vi "CICLO4.vi"() -> ()   [LabVIEW 2013]
panel:
  out "SUMA150":dbl
  out "Contador":dbl
  out "Velocidad Promedio":dbl
  out "Velocidad":dbl(knob) scale=0.0..220.0
  # "GENERAR 10 PRUEBA DE VELOCIDAD\nLUEGO SUMAR LAS VELOCIDADES \nMAYORES A 150 Y OBTENER SU PROMEDIO"
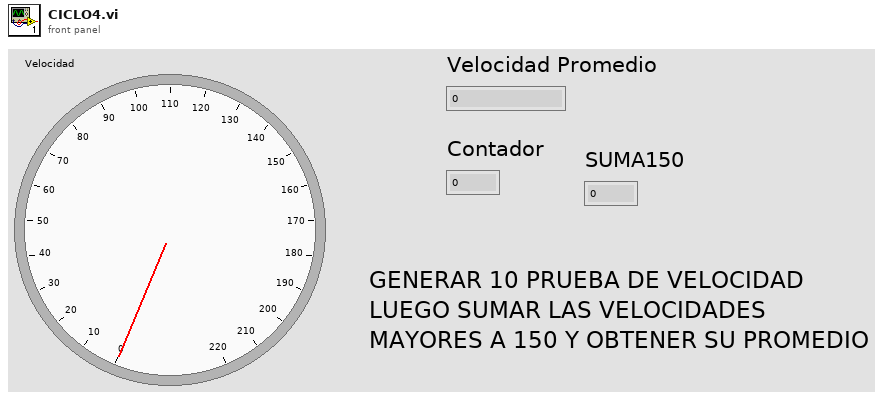
[diagram p1: front panel]
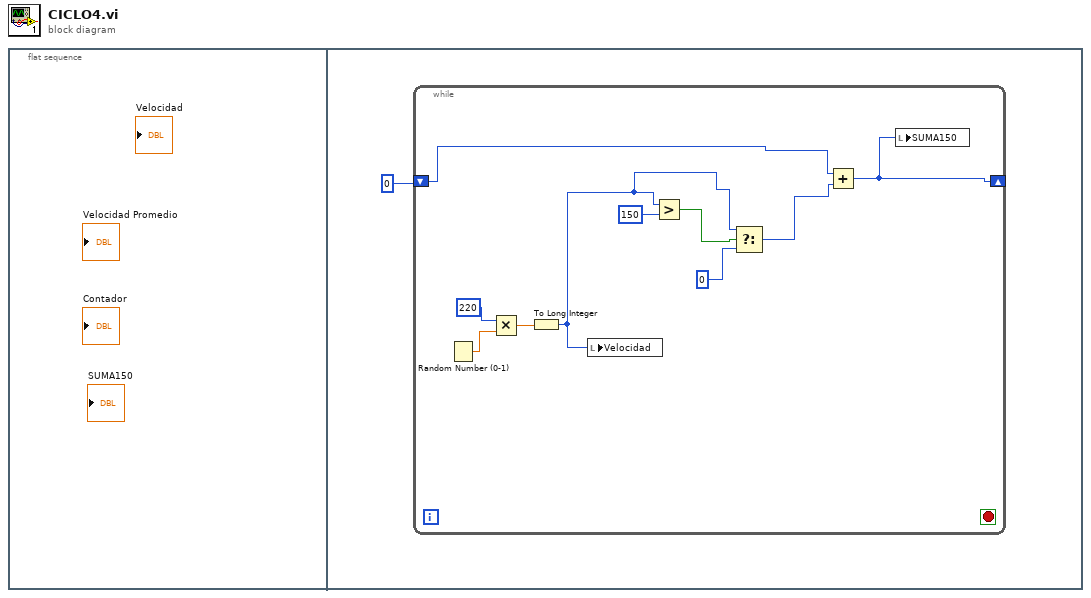
[diagram p0: block diagram]
diagram:
  n1 = flat-sequence {
    frame #0 {
    }
    frame #1 {
      n2 = while {
        shift-right: [w2] -> _
        shift-left: 0 -> [w11]
        stop <- _ stop-if-true
        n3 = Random Number (0-1)() -> (number: 0 to 1=w10:dbl)
        n4 = Multiply(x=220, y=w10) -> (x*y=w8:dbl)
        n5 = To Long Integer(number=w8) -> (32bit integer=w3:i32)
        n6 = local write "Velocidad"(w3) -> ()
        n7 = Greater?(x=w3, y=150) -> (0:w6:bool)
        n8 = Select(t=w3, s=w6, f=0) -> (s? t:f=w4:i32)
        n9 = Add(x=w11, y=w4) -> (x+y=w2:i32)
        n10 = local write "SUMA150"(w2) -> ()
      }
    }
  }
